vi "doAction.vi"(8 "error in (no error)":errorcluster, 10 "ContextData":refnum<class "ContextData.lvclass">, 11 "Initialize in":refnum<class "Launch UI.lvclass">) -> (0 "error out":errorcluster, 2 "ContextData Out":refnum<class "ContextData.lvclass">, 3 "Initialize out":refnum<class "Launch UI.lvclass">)   [LabVIEW 2019, in "Launch UI.lvclass"]
uses:
  Launch UI.lvclass
  ContextData/ContextData.lvclass
panel:
  in  "error in (no error) 2":errorcluster
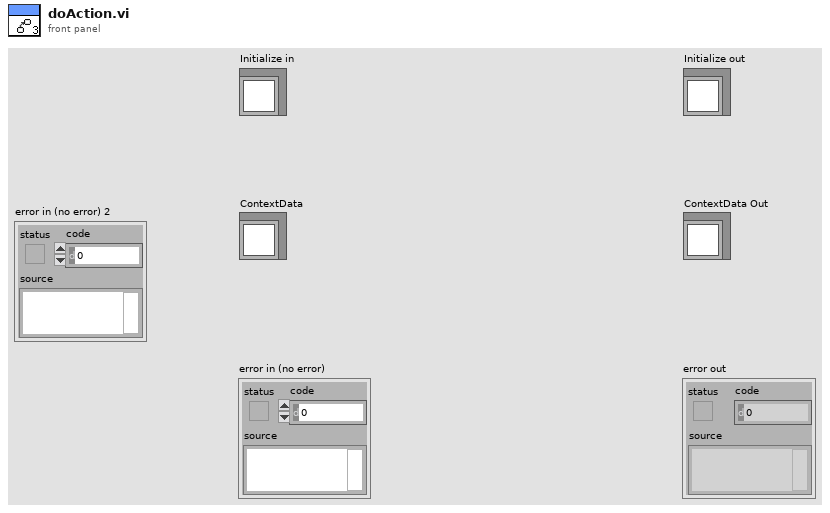
[diagram p1: front panel]
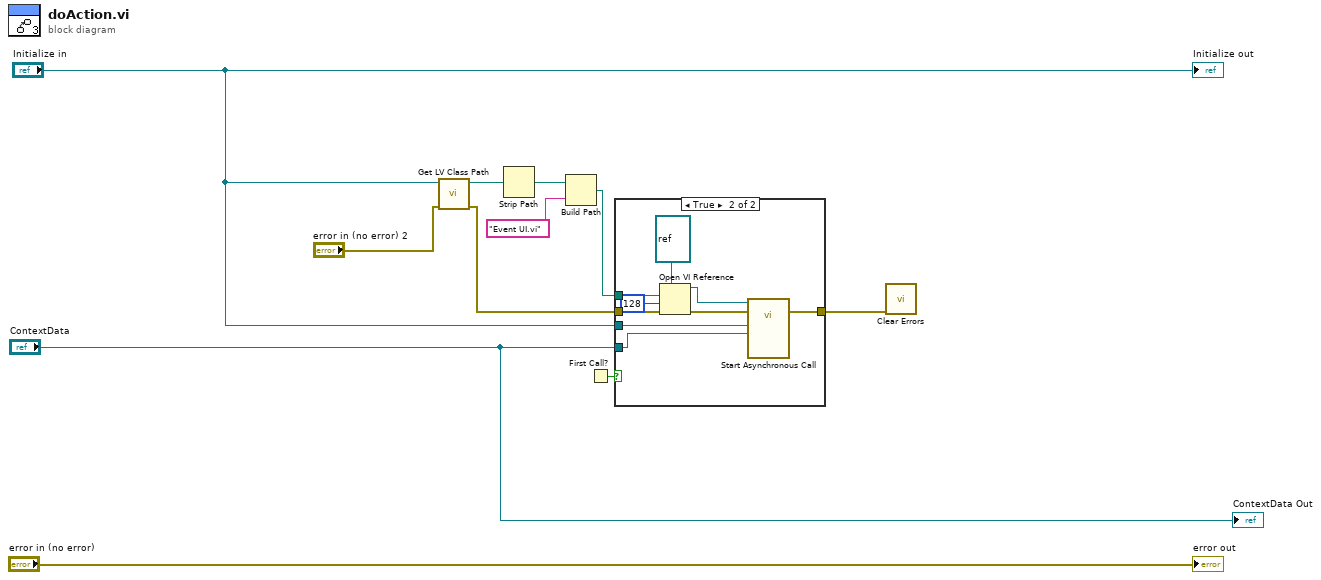
[diagram p0: block diagram]
diagram:
  n1 = call <vilib>:"Get LV Class Path.vi"("error in (no error)"="error in (no error) 2", "object"="Initialize in") -> ("error out"=w8:errorcluster, "class path"=w10:path)  [unwired: 8 in]
  n2 = Strip Path(path=w10) -> (stripped path=w5:path)  [unwired: 1 out]
  n3 = Build Path(base path=w5, name or relative path="Event UI.vi") -> (appended path=w6:path)
  n4 = First Call?() -> (First Call?: T/F=w3:bool)
  n5 = case shown="True" w3 {
    tunnel: w8 -> [w12 w21]
    tunnel: w6 -> [_ w20]
    tunnel: "Initialize in" -> [_ w13]
    tunnel: [w12 w17] -> w4
    tunnel: "ContextData" -> [_ w14]
    frame False {
    }
    frame True {
      n6 = Open VI Reference(type specifier VI Refnum (for type only)=refnum<vi> refnum, vi path=w20, options=128, error in (no error)=w21) -> (vi reference=w16:refnum<vi>, error out=w19:errorcluster)  [unwired: 2 in]
      n7 = call-by-ref "Start Asynchronous Call"(reference=w16, error in=w19, "ContextData In"=w14, "Wait Event in"=w13) -> (error out=w17:errorcluster)  [unwired: 8 in, 3 out]
    }
  }
  n8 = call <vilib>:"Clear Errors.vi"("error in (no error)"=w4) -> ()  [unwired: 5 in, 2 out]
  "error out" <- "error in (no error)"
  "Initialize out" <- "Initialize in"
  "ContextData Out" <- "ContextData"
